vi "4.5.1.vi"   [LabVIEW 2018]
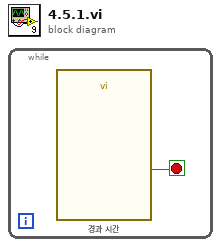
[diagram p0: block diagram]
diagram:
  n1 = while {
    stop <- w1 stop-if-true
    n2 = call "경과 시간"() -> ("Time has Elapsed"=w1:bool)  [unwired: 12 in, 7 out]
  }
